vi "VISA Open.vi"(6 "Serial":T1={"Baud"=9600, "Data Bits"=8, "Parity"=enum."None", "Stop Bits"=10, "Flow"=0, "Term Char?"=TRUE, "Term Char"=10} {"Term Char" format="%02x"; "Flow" items=["None", "XON/XOFF", "RTS/CTS", "XON/XOFF & RTS/CTS", "DTR/DSR", "XON/XOFF & DTR/DSR"]; "Stop Bits" items=["1.0"=10, "1.5"=15, "2.0"=20]}, 7 "Close First? (T)":bool=TRUE, 8 "error in (no error)":errorcluster, 9 "Timeout (10000ms)":u32=10000, 10 "Clear/Flush? (T)":bool=TRUE, 11 "VISA in":refnum<visa-resource-name>) -> (0 "error out":errorcluster, 3 "VISA out":refnum<visa-resource-name>)   [LabVIEW 2018]
uses:
  <vilib>/Instr/_visa.llb/VISA Configure Serial Port (Instr).vi
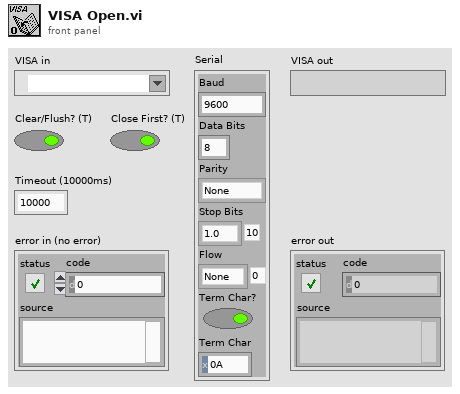
[diagram p1: front panel]
types:
  T1 = cluster{"Baud":u32, "Data Bits":u16, "Parity":enum16{"None", "Odd", "Even", "Mark", "Space"}, "Stop Bits":u16, "Flow":u16, "Term Char?":bool, "Term Char":u8}
  T2 = enum16{"Unknown", "GPIB", "VXI", "GPIB-VXI", "Serial", "PXI", "TCPIP", "USB", "FireWire"}
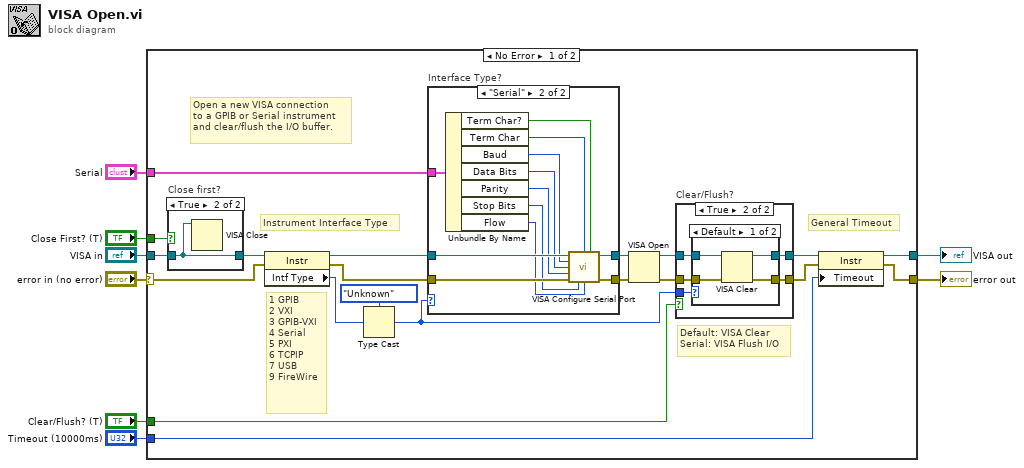
[diagram p0: block diagram]
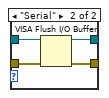
[diagram p4: hidden frame]
diagram:
  n1 = case shown="No Error" "error in (no error)" {
    selector: "error in (no error)" -> [w27 w61]
    tunnel: "VISA in" -> [w11 w60]
    tunnel: "Clear/Flush? (T)" -> [w18 _]
    tunnel: "Serial" -> [w17 _]
    tunnel: [w15 w61] -> w4
    tunnel: [w13 w60] -> w3
    tunnel: "Timeout (10000ms)" -> [w12 _]
    tunnel: "Close First? (T)" -> [w10 _]
    frame No Error {
      # "Open a new VISA connection\nto a GPIB or Serial instrument\nand clear/flush the I/O buffer."
      # "General Timeout"
      # "Default: VISA Clear\nSerial: VISA Flush I/O"
      # "Instrument Interface Type"
      # "1\tGPIB\n2\tVXI\n3\tGPIB-VXI\n4\tSerial\n5\tPXI\n6\tTCPIP\n7\tUSB\n9\tFireWire"
      n2 = case "Close first?" shown="True" w10 {
        tunnel: w11 -> [w29 w30]
        tunnel: [w29 w30] -> w9
        frame False {
        }
        frame True {
          n3 = VISA Close(VISA resource name=w30) -> ()  [unwired: 1 in, 1 out]
        }
      }
      n4 = property class="Instr"(reference=w9, error in=w27) -> (reference out=w25:refnum<visa-resource-name>, error out=w23:errorcluster, "Intf Type"=w28:u16)
      n5 = Type Cast(type=T2."Unknown" ("Interface Type"), x=w28) -> (*(type *) &x=w19:T2)
      n6 = case "Interface Type?" shown="\"Serial\"" w19 {
        tunnel: w25 -> [w47 w59]
        tunnel: [w47 w58] -> w24
        tunnel: w23 -> [w46 w57]
        tunnel: [w46 w56] -> w22
        tunnel: w17 -> [_ w55]
        frame Default {
        }
        frame "Serial" {
          n7 = Unbundle By Name(w55) -> ("Term Char?"=w48:bool, "Term Char"=w49:u8, "Baud"=w54:u32, "Data Bits"=w53:u16, "Parity"=w52:enum16{"None", "Odd", "Even", "Mark", "Space"}, "Stop Bits"=w51:u16, "Flow"=w50:u16)
          n8 = call-poly "VISA Configure Serial Port"("VISA resource name"=w59, "termination char\n(0xA = '\\n' = LF)"=w49, "Enable Termination\nChar (T)"=w48, "baud rate (9600)"=w54, "data bits (8)"=w53, "parity (0:none)"=w52, "error in (no error)"=w57, "stop bits (10: 1 bit)"=w51, "flow control (0:none)"=w50) -> ("VISA resource name out"=w58:refnum<visa-resource-name>, "error out"=w56:errorcluster)  [unwired: 5 in]
        }
      }
      n9 = VISA Open(error in (no error)=w22, VISA resource name=w24) -> (VISA resource name=w21:refnum<visa-resource-name>, error out=w20:errorcluster)  [unwired: 3 in]
      n10 = case "Clear/Flush?" shown="True" w18 {
        tunnel: w21 -> [w32 w37]
        tunnel: [w32 w36] -> w14
        tunnel: w20 -> [w31 w35]
        tunnel: [w31 w34] -> w16
        tunnel: w19 -> [_ w33]
        frame False {
        }
        frame True {
          n11 = case shown="Default" w33 {
            tunnel: w37 -> [w41 w45]
            tunnel: [w38 w44] -> w36
            tunnel: w35 -> [w40 w43]
            tunnel: [w39 w42] -> w34
            frame Default {
              n12 = VISA Clear(VISA resource name=w41, error in (no error)=w40) -> (VISA resource name out=w38:refnum<visa-resource-name>, error out=w39:errorcluster)
            }
            frame "Serial" {
              n13 = VISA Flush I/O Buffer(VISA resource name=w45, error in (no error)=w43) -> (VISA resource name out=w44:refnum<visa-resource-name>, error out=w42:errorcluster)  [unwired: 1 in]
            }
          }
        }
      }
      n14 = property class="Instr"(reference=w14, error in=w16, "Timeout"=w12) -> (reference out=w13:refnum<visa-resource-name>, error out=w15:errorcluster)
    }
    frame Error {
    }
  }
  "VISA out" <- w3
  "error out" <- w4
